vi "sample display.vi"() -> ()   [LabVIEW 2009]
uses:
  display.ctl
panel:
  out "Array":T1[](array[typedef])
  in  "hexadecimal":string
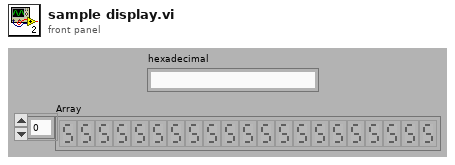
[diagram p1: front panel]
types:
  T1 = typedef "display.ctl" = cluster{"LED 0":bool, "LED 1":bool, "LED 2":bool, "LED 4":bool, "LED 8":bool}
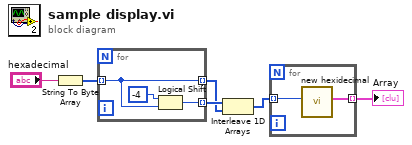
[diagram p0: block diagram]
diagram:
  n1 = String To Byte Array(string="hexadecimal") -> (unsigned byte array=w5:u8[])
  n2 = for {
    tunnel: w5 -> [w7] mode=indexing
    tunnel: [w8] -> w4 mode=indexing
    tunnel: [w7] -> w3 mode=indexing
    n3 = Logical Shift(y=i8 -4, x=w7) -> (x << y=w8:u8)
  }
  n4 = Interleave 1D Arrays(w4, w3) -> (w2:u8[])
  n5 = for {
    tunnel: w2 -> [w11] mode=indexing
    tunnel: [w10] -> w1 mode=indexing
    n6 = call "new hexidecimal.vi"("Numeric"=w11) -> ("display"=w10:T1)  [unwired: 10 in]
  }
  "Array" <- w1
